vi "Actor Core.vi"(8 "error in":errorcluster, 11 "Bioreactor":refnum<class "Bioreactor.lvclass">) -> (0 "error out":errorcluster, 3 "Actor out":refnum<class "Actor.lvclass">)   [LabVIEW 2013, in "Bioreactor.lvlib" / "Bioreactor.lvclass"]
doc: "This is Actor Core.vi, the main message handling loop for Actors. An actor usually just sits in this loop and processes messages as they arrive. Any error returned by the message Do.vi call will stop the loop, with error code 43 as the canonical signal to stop with no error sent to caller. Descendants may override that in Handle Error.vi."
uses:
  Bioreactor.lvclass
  PluginInterface/Actor Framework.lvlibp/Actor/Actor.lvclass
  Bioreactor.lvclass/Bioreactor.ctl
  PluginInterface/PluginInterface.lvlibp/PluginInterfaceClass/PluginInterface.lvclass
  PluginInterface/Actor Framework.lvlibp/Message Enqueuer/Message Priority.ctl
  Write Loop Name.vi
  Write Graph History.vi
  Write Control Value.vi
  Write Control Graph.vi
  Write Process Setpoint.vi
  Write Process Value.vi
  Write Process Graph.vi
  Write Sampling Interval.vi
  PluginInterface/PluginInterface.lvlibp/PluginInterfaceClass/Write VI Refnum.vi
  PluginInterface/Actor Framework.lvlibp/Message Enqueuer/Enqueue.vi
  Bioreactor Messages/Initialize Msg/Initialize Msg.lvclass
  Bioreactor Messages/Read Setpoint Msg/Read Setpoint Msg.lvclass
  Bioreactor Messages/Update Indicators Msg/Update Indicators Msg.lvclass
  Bioreactor Messages/Update Setpoint Msg/Update Setpoint Msg.lvclass
  Bioreactor Messages/Write Setpoint Msg/Write Setpoint Msg.lvclass
  Bioreactor Messages/Read Value Msg/Read Value Msg.lvclass
  Bioreactor Messages/Read Output Msg/Read Output Msg.lvclass
  Bioreactor Messages/Log Data Msg/Log Data Msg.lvclass
  PluginInterface/Actor Framework.lvlibp/Stop Msg/Stop Msg.lvclass
  PluginInterface/Actor Framework.lvlibp/Message Enqueuer/Message Enqueuer.lvclass
panel:
  in  "stop signal":bool
  in  "Sample Interval":i32=1000
  out "Control Value":dbl
  in  "Graph History":dbl=2.0
  in  "Loop Name":u16(ring) caption="View"
  out "Control Graph":T1(graph) caption="Pump A"
  in  "Round Color Box 2":u32(colorbox)=16728642
  in  "Round Color Box":u32(colorbox)=483491
  in  "Process Setpoint":dbl
  out "Proccess Value":dbl
  out "Proccess Graph":T2(graph)
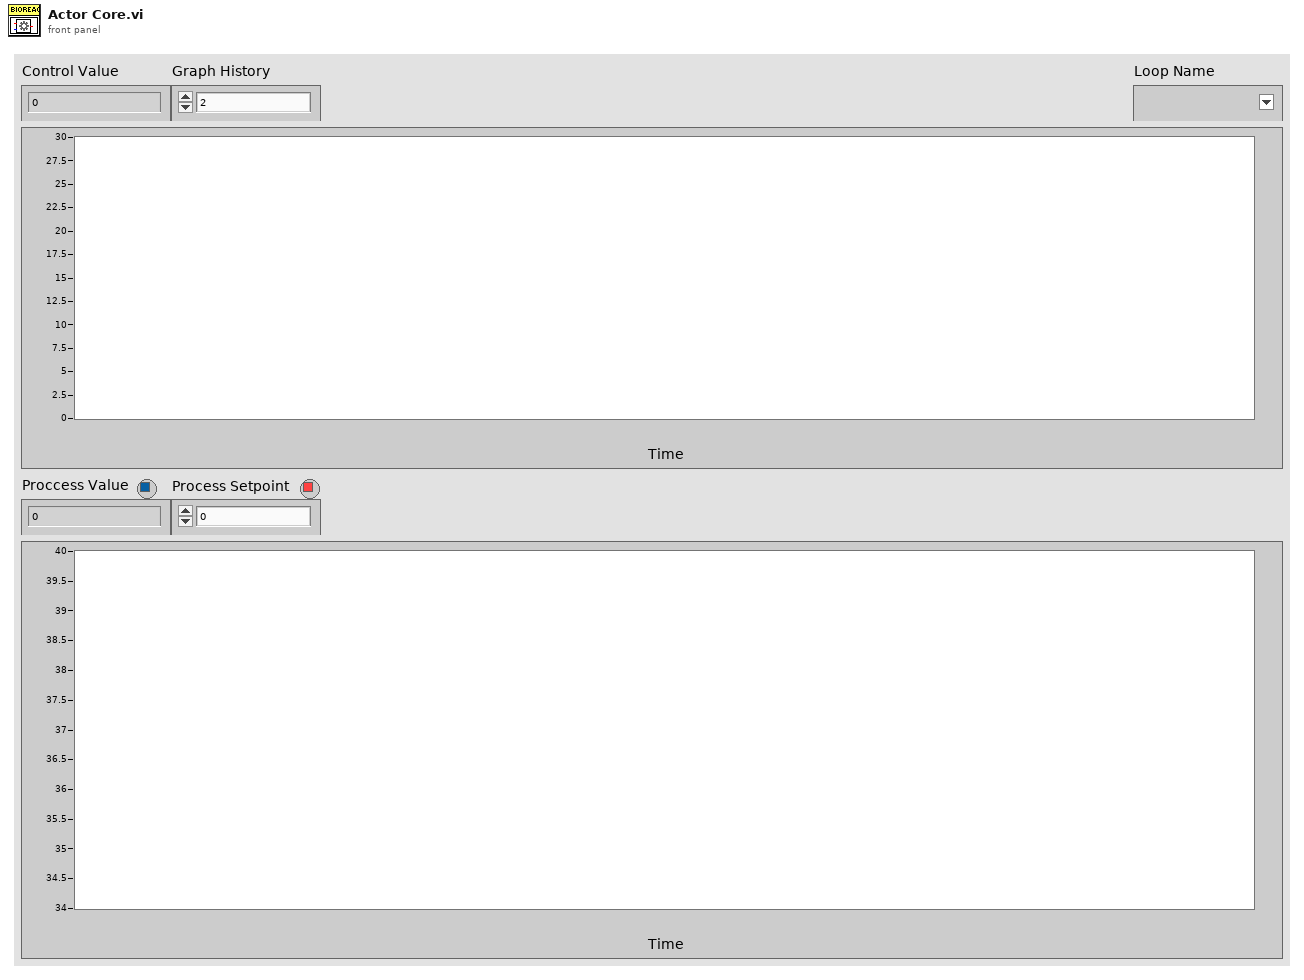
[diagram p1: front panel]
types:
  T1 = cluster{"output array":dbl[], "output array":dbl[]}
  T2 = cluster{"output array":dbl[], "output array":dbl[]}[]
  T3 = typedef "Actor Framework.lvlibp/Message Enqueuer.lvclass/Message Priority.ctl" = enum16{"Low", "Normal", "High"}
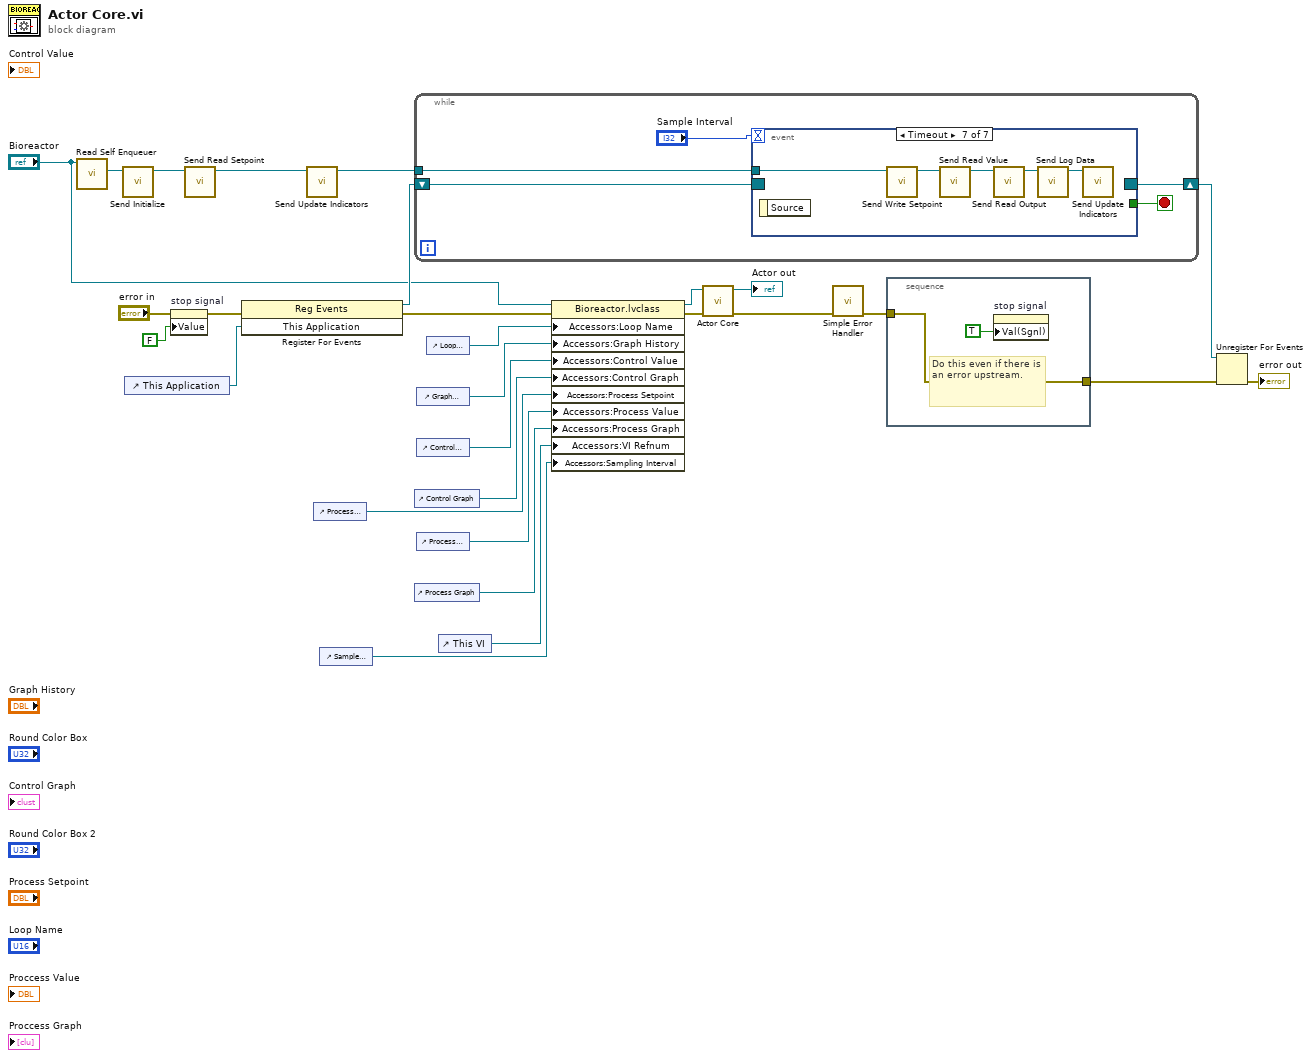
[diagram p0: block diagram]
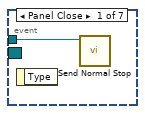
[diagram p2: hidden frame]
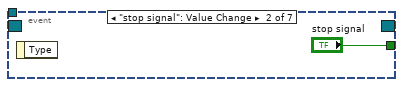
[diagram p3: hidden frame]
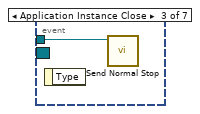
[diagram p4: hidden frame]
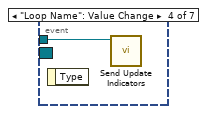
[diagram p5: hidden frame]
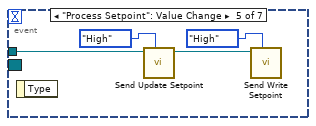
[diagram p6: hidden frame]
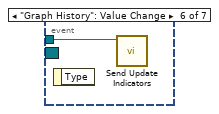
[diagram p7: hidden frame]
diagram:
  n1 = call "Read Self Enqueuer.vi"("Actor"="Bioreactor") -> ("Self Enqueuer"=w7:refnum<class "Message Enqueuer.lvclass">)  [unwired: 10 in]
  n2 = call "Send Initialize.vi"("Message Enqueuer"=w7) -> ("Message Enqueuer out"=w8:refnum<class "Message Enqueuer.lvclass">)  [unwired: 9 in, 1 out]
  n3 = control-ref of="This Application"() -> (w21:refnum<vi>)
  n4 = property on="stop signal" class="Bool (strict)"(error in="error in", "Value"=FALSE ("stop")) -> (error out=w22:errorcluster)  [unwired: 1 in, 1 out]
  n5 = call "Send Read Setpoint.vi"("Message Enqueuer"=w8) -> ("Message Enqueuer out"=w2:refnum<class "Message Enqueuer.lvclass">)  [unwired: 9 in, 1 out]
  n6 = register-events(error in=w22, w21) -> (reference out=w25:refnum<event-registration>, error out=w6:errorcluster)  [unwired: 1 in]
  n7 = call "Send Update Indicators.vi"("Message Enqueuer"=w2) -> ("Message Enqueuer out"=w1:refnum<class "Message Enqueuer.lvclass">)  [unwired: 9 in, 1 out]
  n8 = control-ref of="Process Setpoint"() -> (w13:refnum<vi>)
  n9 = control-ref of="Sample Interval"() -> (w3:refnum<vi>)
  n10 = while {
    tunnel: w1 -> [w33]
    shift-right: [w30] -> w24
    shift-left: w25 -> [w31]
    stop <- w32 stop-if-true
    n11 = event shown="[6] Timeout" {
      selector: w31 -> [_ _ _ _ _ _ _]
      dyn-events: [_ _ _ _ _ _ _] -> w30
      timeout: "Sample Interval" -> [_ _ _ _ _ _ _]
      tunnel: w33 -> [w34 _ w36 w37 w41 w42 w43]
      tunnel: [_ "stop signal" _ _ _ _ _] -> w32
      event Panel Close {
        n12 = event-data() -> ()  [unwired: 1 in, 1 out]
        n13 = call "Send Normal Stop.vi"("Message Enqueuer"=w34) -> ()  [unwired: 10 in, 1 out]
      }
      event "stop signal": Value Change {
        n14 = event-data() -> ()  [unwired: 1 in, 1 out]
      }
      event Application Instance Close {
        n15 = event-data() -> ()  [unwired: 1 in, 1 out]
        n16 = call "Send Normal Stop.vi"("Message Enqueuer"=w36) -> ()  [unwired: 10 in, 1 out]
      }
      event "Loop Name": Value Change {
        n17 = event-data() -> ()  [unwired: 1 in, 1 out]
        n18 = call "Send Update Indicators.vi"("Message Enqueuer"=w37) -> ()  [unwired: 9 in, 2 out]
      }
      event "Process Setpoint": Value Change {
        n19 = event-data() -> ()  [unwired: 1 in, 1 out]
        n20 = call "Send Update Setpoint.vi"("Message Priority (Normal)"=Message_Priority."High", "Message Enqueuer"=w41) -> ("Message Enqueuer out"=w40:refnum<class "Message Enqueuer.lvclass">)  [unwired: 8 in, 1 out]
        n21 = call "Send Write Setpoint.vi"("Message Priority (Normal)"=Message_Priority."High", "Message Enqueuer"=w40) -> ()  [unwired: 8 in, 2 out]
      }
      event "Graph History": Value Change {
        n22 = event-data() -> ()  [unwired: 1 in, 1 out]
        n23 = call "Send Update Indicators.vi"("Message Enqueuer"=w42) -> ()  [unwired: 9 in, 2 out]
      }
      event Timeout {
        n24 = event-data() -> ()  [unwired: 1 in, 1 out]
        n25 = call "Send Write Setpoint.vi"("Message Enqueuer"=w43) -> ("Message Enqueuer out"=w44:refnum<class "Message Enqueuer.lvclass">)  [unwired: 9 in, 1 out]
        n26 = call "Send Read Value.vi"("Message Enqueuer"=w44) -> ("Message Enqueuer out"=w47:refnum<class "Message Enqueuer.lvclass">)  [unwired: 9 in, 1 out]
        n27 = call "Send Read Output.vi"("Message Enqueuer"=w47) -> ("Message Enqueuer out"=w46:refnum<class "Message Enqueuer.lvclass">)  [unwired: 9 in, 1 out]
        n28 = call "Send Log Data.vi"("Message Enqueuer"=w46) -> ("Message Enqueuer out"=w45:refnum<class "Message Enqueuer.lvclass">)  [unwired: 9 in, 1 out]
        n29 = call "Send Update Indicators.vi"("Message Enqueuer"=w45) -> ()  [unwired: 9 in, 2 out]
      }
    }
  }
  n30 = control-ref of="Control Graph"() -> (w14:refnum<vi>)
  n31 = control-ref of="Process Graph"() -> (w11:refnum<vi>)
  n32 = control-ref of="Graph History"() -> (w15:refnum<vi>)
  n33 = control-ref of="Control Value"() -> (w9:refnum<vi>)
  n34 = control-ref of="Process Value"() -> (w12:refnum<vi>)
  n35 = control-ref of="Loop Name"() -> (w5:refnum<vi>)
  n36 = control-ref of="This VI"() -> (w10:refnum<vi>)
  n37 = property class="Bioreactor.lvclass"(reference="Bioreactor", error in=w6, "Accessors:Loop Name"=w5, "Accessors:Graph History"=w15, "Accessors:Control Value"=w9, "Accessors:Control Graph"=w14, "Accessors:Process Setpoint"=w13, "Accessors:Process Value"=w12, "Accessors:Process Graph"=w11, "Accessors:VI Refnum"=w10, "Accessors:Sampling Interval"=w3) -> (reference out=w19:refnum<class "Bioreactor.lvclass">, error out=w20:errorcluster)
  n38 = call-parent "Actor Core.vi"("error in"=w20, "Actor in"=w19) -> ("error out"=w27:errorcluster, "Actor out"=→"Actor out":refnum<class "Actor.lvclass">)  [unwired: 8 in]
  n39 = call <vilib>:"Simple Error Handler.vi"("error in (no error)"=w27) -> ("error out"=w26:errorcluster)  [unwired: 4 in, 4 out]
  n40 = stacked-sequence {
    tunnel: [w48] -> w23
    tunnel: w26 -> [w48]
    frame #0 {
      # "Do this even if there is an error upstream."
      n41 = property on="stop signal" class="Bool (strict)"("Val(Sgnl)"=TRUE ("stop")) -> ()  [unwired: 2 in, 2 out]
    }
  }
  n42 = Unregister For Events(event registration refnum=w24, error in=w23) -> (error out=→"error out":errorcluster)
